vi "acel_processing.vi"(7 "rate":dbl, 8 "error in":errorcluster, 11 "acelData":dbl[][](array[numeric])) -> (0 "error out":errorcluster, 3 "RMS":dbl[](array[numeric]))   [LabVIEW 2016]
uses:
  <vilib>/Analysis/5stat.llb/RMS (DBL).vi
  <vilib>/Analysis/NI_AALPro.lvlib
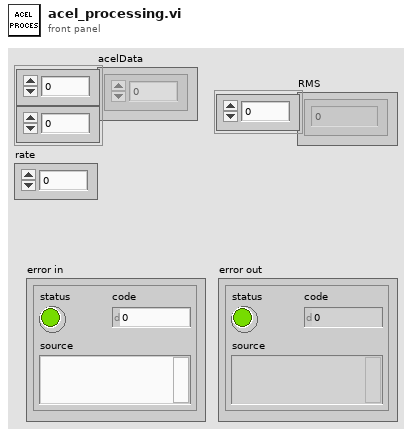
[diagram p1: front panel]
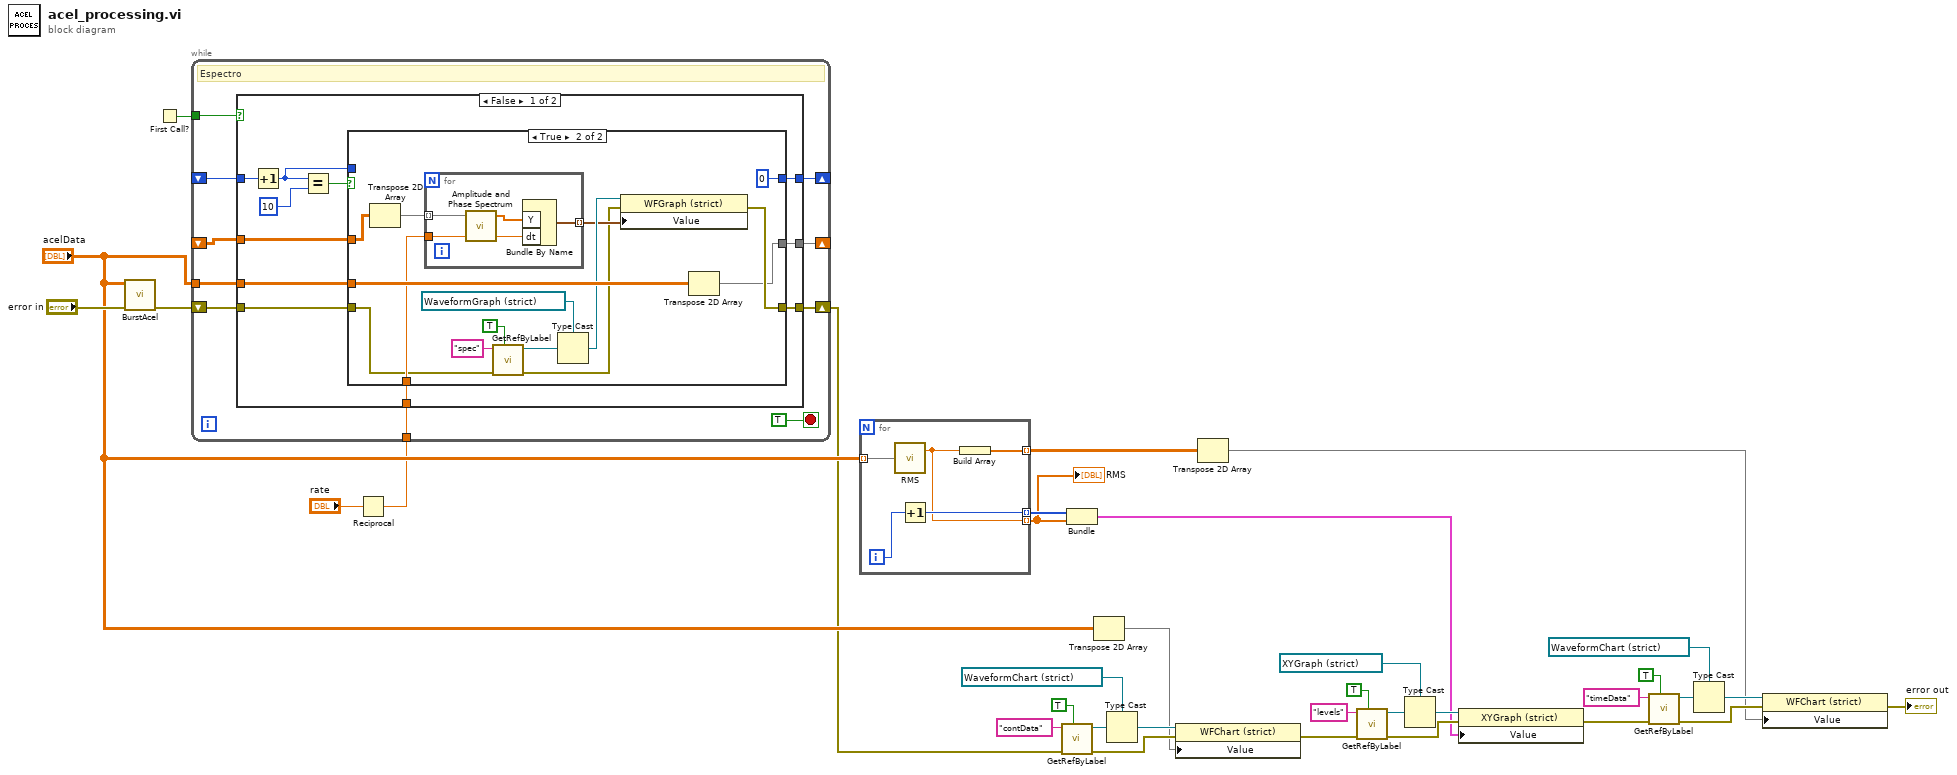
[diagram p0: block diagram]
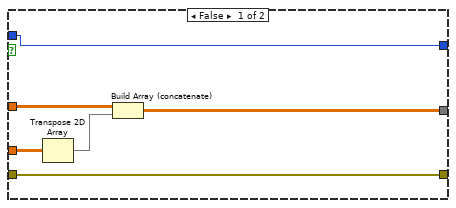
[diagram p2: hidden frame]
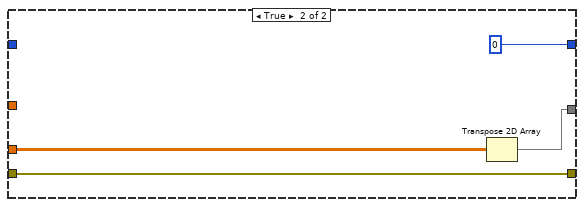
[diagram p3: hidden frame]
diagram:
  n1 = call "BurstAcel.vi"("error in"="error in", "acelData"="acelData") -> ("error out"=w5:errorcluster)  [unwired: 9 in]
  n2 = First Call?() -> (First Call?: T/F=w4:bool)
  n3 = Reciprocal(x="rate") -> (1/x=w3:dbl)
  n4 = while {
    shift-right: [w43] -> _
    shift-left: _ -> [w42]
    shift-right: [w39] -> w2
    shift-left: w5 -> [w41]
    tunnel: "acelData" -> [w40]
    tunnel: w4 -> [w38]
    shift-right: [w37] -> _
    shift-left: _ -> [w36]
    tunnel: w3 -> [w35]
    stop <- TRUE stop-if-true
    # "Espectro"
    n5 = case shown="False" w38 {
      tunnel: [w52 0] -> w43
      tunnel: w42 -> [w55 _]
      tunnel: w41 -> [w51 w84]
      tunnel: w40 -> [w50 w83]
      tunnel: [w49 w84] -> w39
      tunnel: [w47 w82] -> w37
      tunnel: w36 -> [w46 _]
      tunnel: w35 -> [w45 _]
      frame False {
        n6 = Increment(x=w55) -> (x+1=w48:i32)
        n7 = Equal?(x=w48, y=10) -> (x = y?=w53:bool)
        n8 = case shown="True" w53 {
          tunnel: [w61 0 ("y")] -> w52
          tunnel: w51 -> [w60 w70]
          tunnel: w50 -> [w58 w75]
          tunnel: [w60 w64] -> w49
          tunnel: w48 -> [w61 _]
          tunnel: [w56 w62] -> w47
          tunnel: w46 -> [w59 w74]
          tunnel: w45 -> [_ w73]
          frame False {
            n9 = Transpose 2D Array(2D array=w58) -> (transposed array=w57:dbl[][])
            n10 = Build Array (concatenate)(w59, w57) -> (w56:dbl[][])
          }
          frame True {
            n11 = Transpose 2D Array(2D array=w74) -> (transposed array=w63:dbl[][])
            n12 = for {
              tunnel: w63 -> [w79] mode=indexing
              tunnel: w73 -> [w78]
              tunnel: [w77] -> w66 mode=indexing
              n13 = call <vilib>:"Amplitude and Phase Spectrum.vi"("dt"=w78, "Signal (V)"=w79) -> ("df"=w81:dbl, "Amp Spectrum Mag (Vrms)"=w80:dbl[])  [unwired: 1 in, 1 out]
              n14 = Bundle By Name("Y"=w80, "dt"=w81) -> (w77:waveform(dbl))  [unwired: 1 in]
            }
            n15 = call "GetRefByLabel.vi"("InsideTab"=TRUE, "error in"=w70, "Label"="spec") -> ("error out"=w65:errorcluster, "Ctl Refnum"=w71:refnum<vi>)  [unwired: 6 in, 1 out]
            n16 = Type Cast(type=refnum<vi> refnum ("spec"), x=w71) -> (*(type *) &x=w67:refnum<vi>)
            n17 = property class="WFGraph (strict)"(reference=w67, error in=w65, "Value"=w66) -> (error out=w64:errorcluster)  [unwired: 1 out]
            n18 = Transpose 2D Array(2D array=w75) -> (transposed array=w62:dbl[][])
          }
        }
      }
      frame True {
        n19 = Transpose 2D Array(2D array=w83) -> (transposed array=w82:dbl[][])
      }
    }
  }
  n20 = for {
    tunnel: "acelData" -> [w86] mode=indexing
    tunnel: [w89] -> w20 mode=indexing
    tunnel: [w88] -> w34 mode=indexing
    tunnel: [w87] -> w9 mode=indexing
    i -> [w90]
    n21 = call-poly <vilib>:"RMS.vi"("X"=w86) -> ("rms value"=w87:dbl)  [unwired: 1 out]
    n22 = Increment(x=w90) -> (x+1=w88:i32)
    n23 = Build Array(w87) -> (w89:dbl[])
  }
  "RMS" <- w9
  n24 = call "GetRefByLabel.vi"("InsideTab"=TRUE, "error in"=w2, "Label"="contData") -> ("error out"=w14:errorcluster, "Ctl Refnum"=w15:refnum<vi>)  [unwired: 6 in, 1 out]
  n25 = Bundle(w34, w9) -> (w28:cluster{i32[], dbl[]})  [unwired: 1 in]
  n26 = Transpose 2D Array(2D array="acelData") -> (transposed array=w10:dbl[][])
  n27 = Type Cast(type=refnum<vi> refnum ("timeData"), x=w15) -> (*(type *) &x=w16:refnum<vi>)
  n28 = property class="WFChart (strict)"(reference=w16, error in=w14, "Value"=w10) -> (error out=w11:errorcluster)  [unwired: 1 out]
  n29 = Transpose 2D Array(2D array=w20) -> (transposed array=w1:dbl[][])
  n30 = call "GetRefByLabel.vi"("InsideTab"=TRUE, "error in"=w11, "Label"="levels") -> ("error out"=w29:errorcluster, "Ctl Refnum"=w31:refnum<vi>)  [unwired: 6 in, 1 out]
  n31 = Type Cast(type=refnum<vi> refnum ("levels"), x=w31) -> (*(type *) &x=w30:refnum<vi>)
  n32 = property class="XYGraph (strict)"(reference=w30, error in=w29, "Value"=w28) -> (error out=w25:errorcluster)  [unwired: 1 out]
  n33 = call "GetRefByLabel.vi"("InsideTab"=TRUE, "error in"=w25, "Label"="timeData") -> ("error out"=w23:errorcluster, "Ctl Refnum"=w22:refnum<vi>)  [unwired: 6 in, 1 out]
  n34 = Type Cast(type=refnum<vi> refnum ("timeData"), x=w22) -> (*(type *) &x=w21:refnum<vi>)
  n35 = property class="WFChart (strict)"(reference=w21, error in=w23, "Value"=w1) -> (error out=→"error out":errorcluster)  [unwired: 1 out]
